vi "slope.vi"(8 "y 2":dbl, 9 "y1":dbl, 10 "x 2":dbl, 11 "x1":dbl) -> (2 "Slope":dbl)   [LabVIEW 2012]
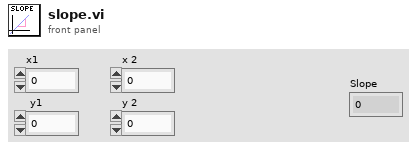
[diagram p1: front panel]
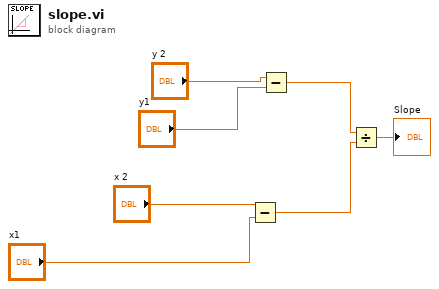
[diagram p0: block diagram]
diagram:
  n1 = Subtract(x="x 2", y="x1") -> (x-y=w2:dbl)
  n2 = Subtract(x="y 2", y="y1") -> (x-y=w3:dbl)
  n3 = Divide(x=w3, y=w2) -> (x/y=→"Slope":dbl)
